vi "DAQmx Start Trigger (None).vi"(0 "task/channels in":refnum<k21>, 11 "error in":errorcluster) -> (4 "task out":refnum<k21>, 15 "error out":errorcluster)   [LabVIEW 2020]
doc: "Configures the task to start acquiring or generating samples immediately upon starting the task."
uses:
  nilvaiu.dll
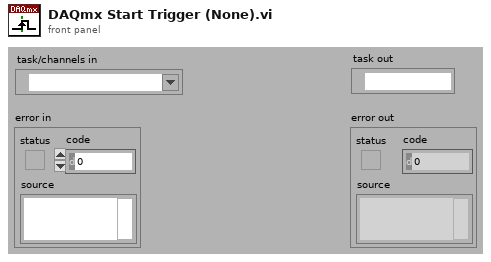
[diagram p1: front panel]
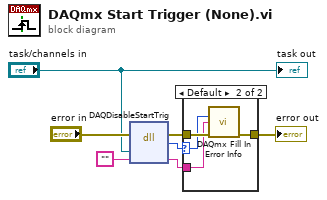
[diagram p0: block diagram]
diagram:
  n1 = dll-call lib="nilvaiu.*" fn="DAQDisableStartTrig"(error in="error in", "taskID"="task/channels in", "extendedErrorIndo"="") -> (error out=w4:errorcluster, "return type"=w2:i32, "extendedErrorIndo"=w3:string)  [unwired: 3 in, 1 out]
  n2 = case shown="Default" w2 {
    selector: w2 -> [_ w10]
    tunnel: w4 -> [w8 w12]
    tunnel: [w8 w11] -> w6
    tunnel: w3 -> [_ w9]
    frame 0 {
    }
    frame Default {
      n3 = call "DAQmx Fill In Error Info.vi"("status code"=w10, "extended error info"=w9, "error in"=w12) -> ("error out"=w11:errorcluster)  [unwired: 1 in, 11 out]
    }
  }
  "error out" <- w6
  "task out" <- "task/channels in"
